vi "RegisteredMessages.vi"() -> (3 "registered messages":string[](array[string]))   [LabVIEW 2017, in "TestPanel.lvlib"]
uses:
  <vilib>/addons/InsightCM/Devices/Shared/Common/TestPanel/TestPanel.lvlib
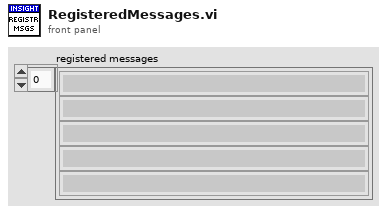
[diagram p1: front panel]
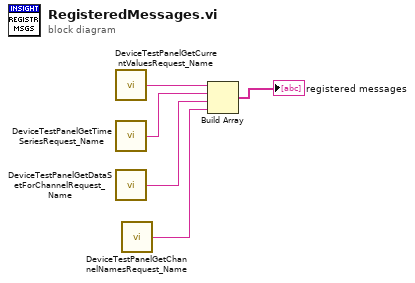
[diagram p0: block diagram]
diagram:
  n1 = call <vilib>:"DeviceTestPanelGetCurrentValuesRequest_Name.vi"() -> ("MessageName"=w4:string)  [unwired: 5 in]
  n2 = call <vilib>:"DeviceTestPanelGetTimeSeriesRequest_Name.vi"() -> ("MessageName"=w3:string)  [unwired: 5 in]
  n3 = call <vilib>:"DeviceTestPanelGetDataSetForChannelRequest_Name.vi"() -> ("MessageName"=w2:string)  [unwired: 5 in]
  n4 = call <vilib>:"DeviceTestPanelGetChannelNamesRequest_Name.vi"() -> ("MessageName"=w1:string)  [unwired: 5 in]
  n5 = Build Array(w4, w3, w2, w1) -> (→"registered messages":string[])
